vi "osa_create data file.vi"(8 "error in (no error)":errorcluster, 9 "column headers":string[](array[string])=["ms_timer", "teensy_timer", "code", "bus_num", "osb_index", "sensor_index", "sensor_ID", "data_1", "data_2", "valid"], 11 "data folder in":path) -> (0 "error out":errorcluster, 1 "status string":string, 2 "data file refnum":refnum<file>, 3 "data folder out":path)   [LabVIEW 2021]
uses:
  <vilib>/Utility/error.llb/whitespace.ctl
panel:
  # "OSA subVI: create data file with time stamp in file name, write column headers"
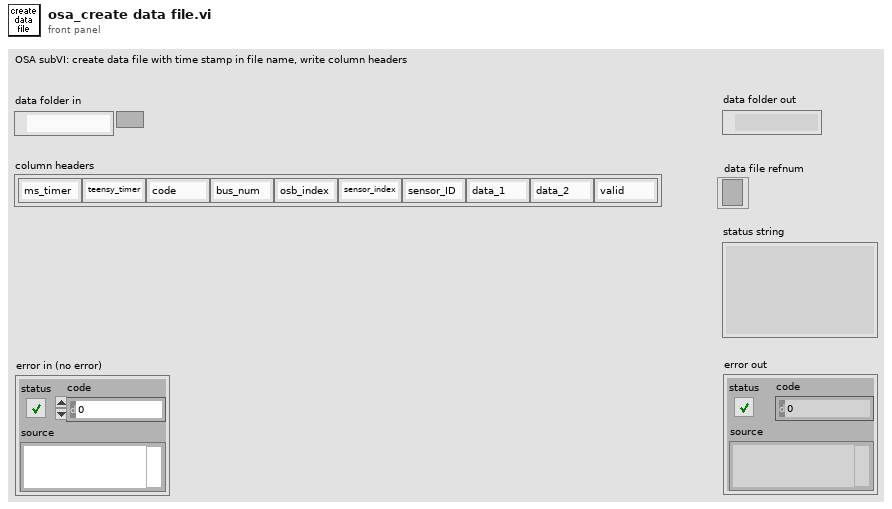
[diagram p1: front panel]
types:
  T1 = typedef "whitespace.ctl" = u16
  T2 = enum16{"open", "replace", "create", "open or create", "replace or create", "replace or create with confirmation"}
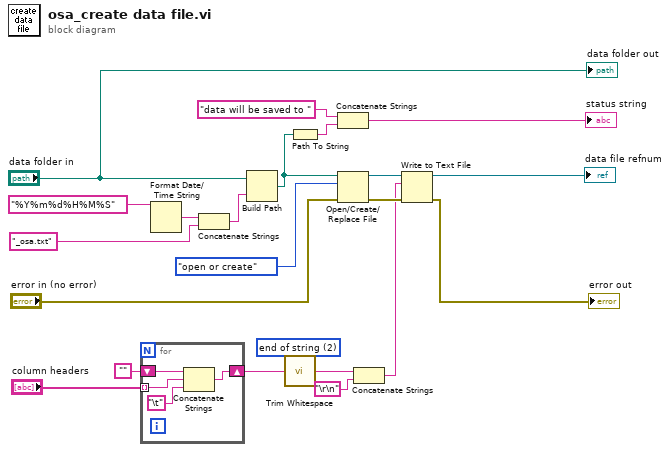
[diagram p0: block diagram]
diagram:
  w3 = T1 2 items=["both", "start of string", "end of string"] ("location (both)")
  n1 = for {
    tunnel: "column headers" -> [w25] mode=indexing
    shift-right: [w24] -> w1
    shift-left: "" -> [w26]
    n2 = Concatenate Strings(w26, w25, "\t") -> (w24:string)
  }
  n3 = Format Date/Time String(time format string (%c)="%Y%m%d%H%M%S") -> (date/time string=w21:string)  [unwired: 2 in]
  n4 = Concatenate Strings(w21, "_osa.txt") -> (w19:string)
  n5 = Build Path(base path="data folder in", name or relative path=w19) -> (appended path=w16:path)
  n6 = call <vilib>:"Trim Whitespace.vi"("string"=w1, "location (both)"=w3) -> ("trimmed string"=w2:string)
  n7 = Path To String(path=w16) -> (string=w15:string)
  n8 = Concatenate Strings("data will be saved to ", w15) -> (→"status string":string)
  n9 = Open/Create/Replace File(file path (use dialog)=w16, error in="error in (no error)", operation (0:open)=T2."open or create") -> (refnum out=w11:refnum<file>, error out=w10:errorcluster)  [unwired: 3 in, 1 out]
  n10 = Concatenate Strings(w2, "\r\n") -> (w4:string)
  n11 = Write to Text File(file (use dialog)=w11, text=w4, error in=w10) -> (refnum out=→"data file refnum":refnum<file>, error out=→"error out":errorcluster)  [unwired: 1 in, 1 out]
  "data folder out" <- "data folder in"
